vi "PWM Output.vi"() -> ()   [LabVIEW 2025]
panel:
  out "error out":errorcluster
  in  "Duty Cycle":u8(slide) scale=0.0..255.0
  in  "Pin_PWM":u8=4 min=4 max=40
  in  "VISA resource name":refnum<visa-resource-name>
  in  "stop":bool
  # "Ejemplo: Control de PWM\nEste ejemplo muestra cómo generar una señal PWM (Pulse Width Modulation) en LV_ESP32, permitiendo controlar el ciclo de trabajo de un pin de salida para manejar dispositivos como motores, LEDs o actuadores.\n\nEntradas requeridas:\nPin_PWM: Pin en el que se generará la señal PWM.\nDuty Cycle: Valor que define el ciclo de trabajo de la señal (0-255).\n\nSalidas generadas:\nSeñal PWM física aplicada en el pin configurado."
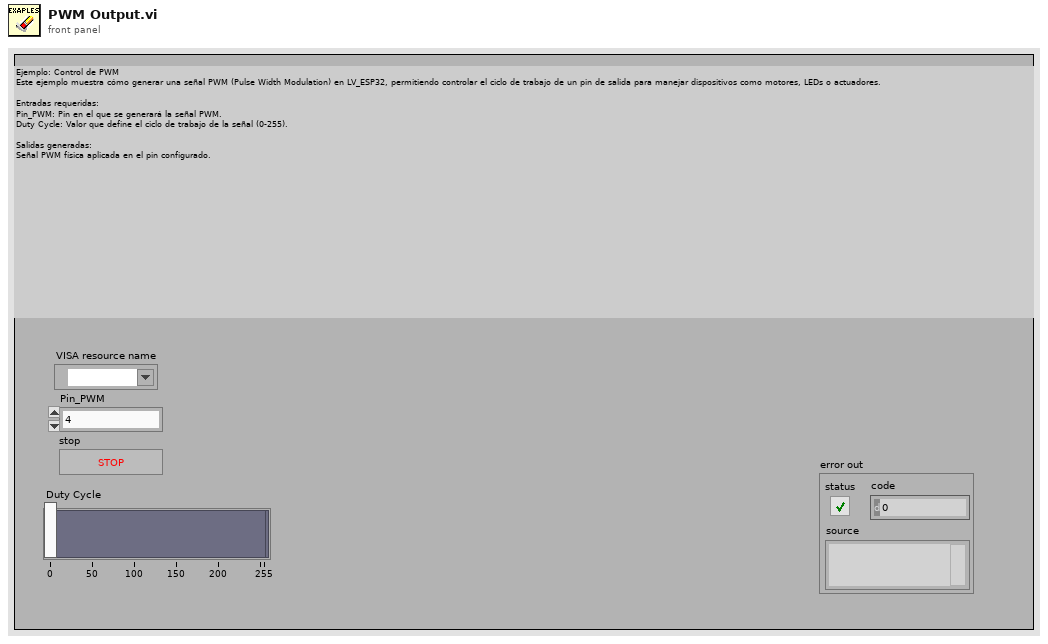
[diagram p1: front panel]
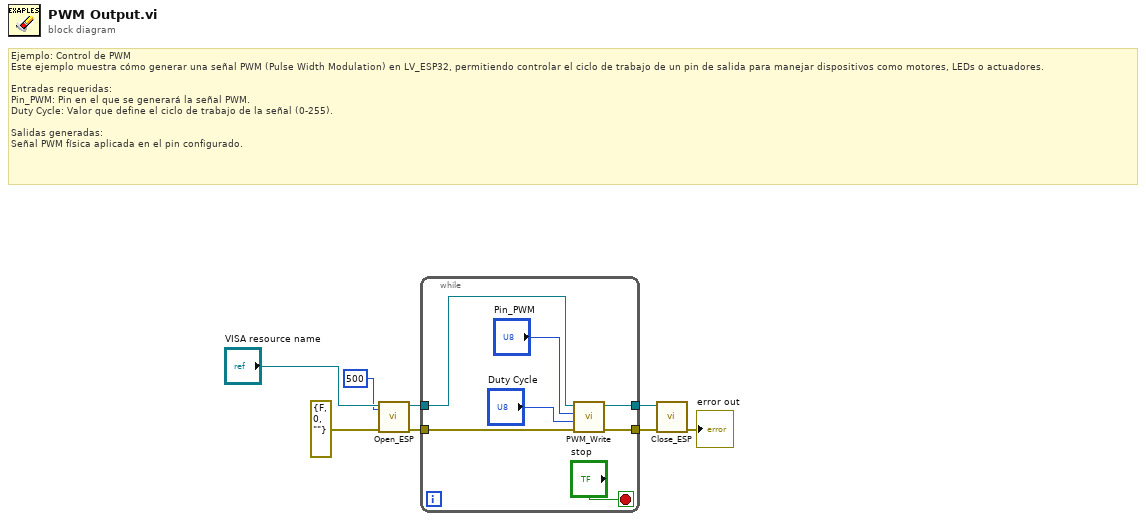
[diagram p0: block diagram]
diagram:
  # "Ejemplo: Control de PWM\nEste ejemplo muestra cómo generar una señal PWM (Pulse Width Modulation) en LV_ESP32, permitiendo controlar el ciclo de trabajo de un pin de salida para manejar dispositivos como motores, LEDs o actuadores.\n\nEntradas requeridas:\nPin_PWM: Pin en el que se generará la señal PWM.\nDuty Cycle: Valor que define el ciclo de trabajo de la señal (0-255).\n\nSalidas generadas:\nSeñal PWM física aplicada en el pin configurado."
  n1 = call "Open_ESP.vi"("timeout (10sec)"=u32 500, "error in (no error)"=errorcluster {"status"=FALSE, "code"=0, "source"=""}, "VISA resource name"="VISA resource name") -> ("error out"=w6:errorcluster, "VISA resource name out"=w5:refnum<visa-resource-name>)  [unwired: 7 in]
  n2 = while {
    tunnel: [w14] -> w8
    tunnel: [w13] -> w7
    tunnel: w6 -> [w12]
    tunnel: w5 -> [w11]
    stop <- "stop" stop-if-true
    n3 = call "PWM_Write.vi"("error in (no error)"=w12, "DC"="Duty Cycle", "Pin"="Pin_PWM", "VISA resource name"=w11) -> ("error out"=w13:errorcluster, "VISA resource name out"=w14:refnum<visa-resource-name>)  [unwired: 6 in]
  }
  n4 = call "Close_ESP.vi"("error in (no error)"=w7, "VISA resource name"=w8) -> ("error out"=→"error out":errorcluster)  [unwired: 9 in]
